vi "Actor Core.vi"(8 "error in":errorcluster, 11 "Project View in":refnum<class "Project View.lvclass">) -> (0 "error out":errorcluster, 3 "Actor out":refnum<class "Actor.lvclass">)   [LabVIEW 2013, in "SET Project Editor.lvlib" / "Project View.lvclass"]
doc: "(<B>Filename</B>: Actor Framework.lvlib:Actor.lvclass:Actor Core.vi)\n\nReceives messages to the actor, reacts to them, and initiates any error handling that may shut the actor down.\n\nDescendant classes may override this VI to append parallel tasks for the actor to complete while it handles messages. Overrides use the Call Parent Method node."
uses:
  Project View.lvclass
  <vilib>/ActorFramework/Actor/Actor.lvclass
  <vilib>/ActorFramework/Actor/Actor.lvclass/Actor.ctl
  <vilib>/ActorFramework/Message Enqueuer/Message Enqueuer.lvclass/Message Enqueuer.ctl
  UI View/UI View.lvclass
  <vilib>/ActorFramework/Message Enqueuer/Init from Existing Queue.vi
  <vilib>/ActorFramework/Message Enqueuer/Message Enqueuer.lvclass
panel:
  # "SET Localization Project Editor"
  # "Version 0.3.8"
  # "Copyright © 2014, Ryan Porter. All rights reserved."
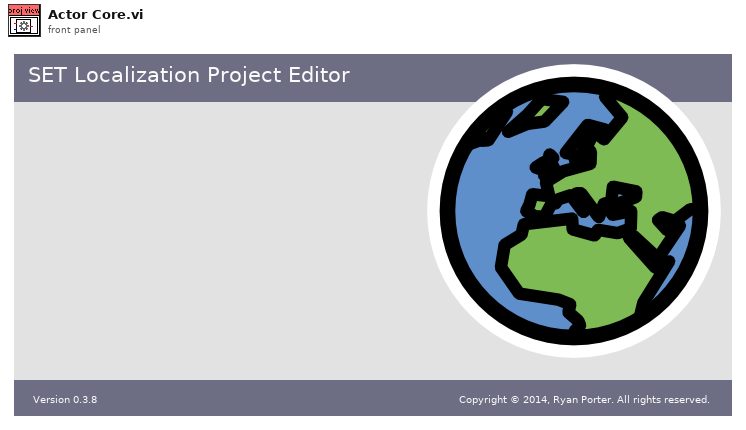
[diagram p1: front panel]
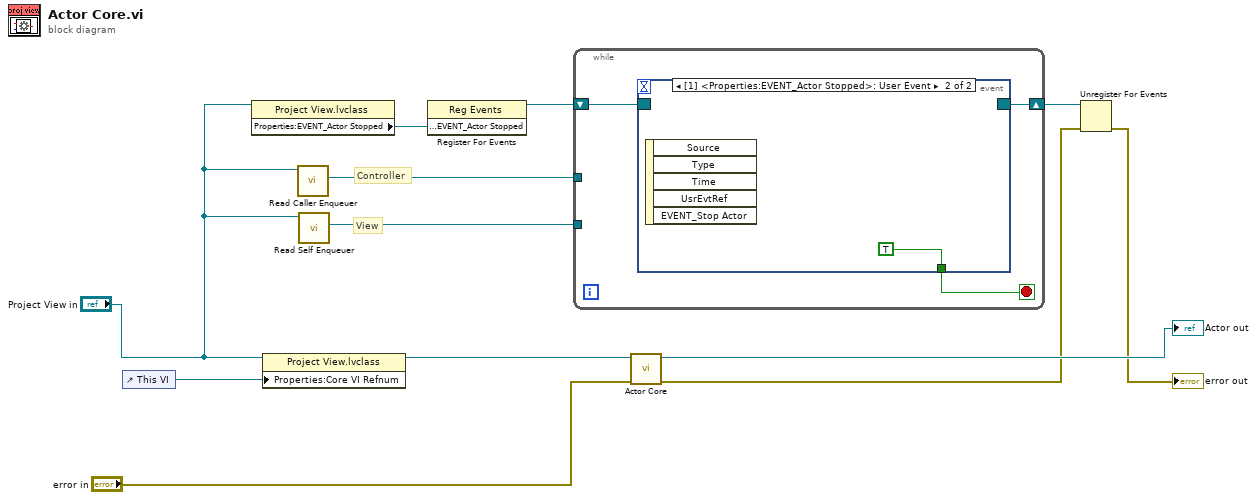
[diagram p0: block diagram]
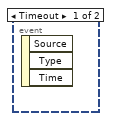
[diagram p2: hidden frame]
diagram:
  # "Controller"
  # "View"
  n1 = control-ref of="This VI"() -> (w1:refnum<vi>)
  n2 = property class="Project View.lvclass"(reference="Project View in") -> ("Properties:EVENT_Actor Stopped"=w8:refnum<user-event>)  [unwired: 1 in, 2 out]
  n3 = property class="Project View.lvclass"(reference="Project View in", "Properties:Core VI Refnum"=w1) -> (reference out=w2:refnum<class "Project View.lvclass">)  [unwired: 1 in, 1 out]
  n4 = call <vilib>:"Read Caller Enqueuer.vi"("Actor"="Project View in") -> ("Caller Enqueuer"=w10:refnum<class "Message Enqueuer.lvclass">)  [unwired: 10 in]
  n5 = call <vilib>:"Read Self Enqueuer.vi"("Actor"="Project View in") -> ("Self Enqueuer"=w9:refnum<class "Message Enqueuer.lvclass">)  [unwired: 10 in]
  n6 = register-events(w8) -> (reference out=w7:refnum<event-registration>)  [unwired: 2 in, 1 out]
  n7 = while {
    tunnel: w10 -> [_]
    tunnel: w9 -> [_]
    shift-right: [w13] -> w6
    shift-left: w7 -> [w15]
    stop <- w14 stop-if-true
    n8 = event shown="[1] <Properties:EVENT_Actor Stopped>: User Event" {
      selector: w15 -> [_ _]
      dyn-events: [_ _] -> w13
      timeout: _ -> [_ _]
      tunnel: [_ TRUE] -> w14
      event Timeout {
        n9 = event-data() -> ()  [unwired: 1 in, 3 out]
      }
      event User Event {
        n10 = event-data() -> ()  [unwired: 1 in, 5 out]
      }
    }
  }
  n11 = call-parent "Actor Core.vi"("error in"="error in", "Actor in"=w2) -> ("error out"=w5:errorcluster, "Actor out"=→"Actor out":refnum<class "Actor.lvclass">)  [unwired: 8 in]
  n12 = Unregister For Events(event registration refnum=w6, error in=w5) -> (error out=→"error out":errorcluster)
